vi "NIVEL DE TANQUE.vi"() -> ()   [LabVIEW 2019]
panel:
  in  "Velocidad de Llenado":dbl(knob) scale=0.0..10.0
  in  "Accion":bool
  in  "Vaciado/Llenado":bool
  in  "Velocidad":bool
  out "Tanque Vacio":bool
  out "Tanque LLeno":bool
  out "Paro":bool
  out "Vaciando":bool
  out "Llenando":bool
  out "Tanque":dbl(slide) scale=0.0..1000.0
  # "LLENAR"
  # "VACIAR"
  # "ALTA"
  # "CONTINUAR"
  # "PARAR"
  # "BAJA"
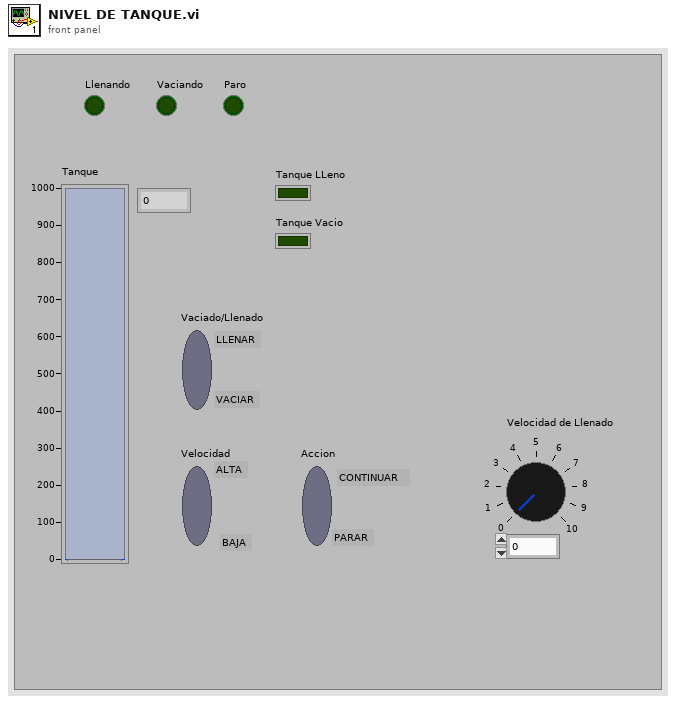
[diagram p1: front panel]
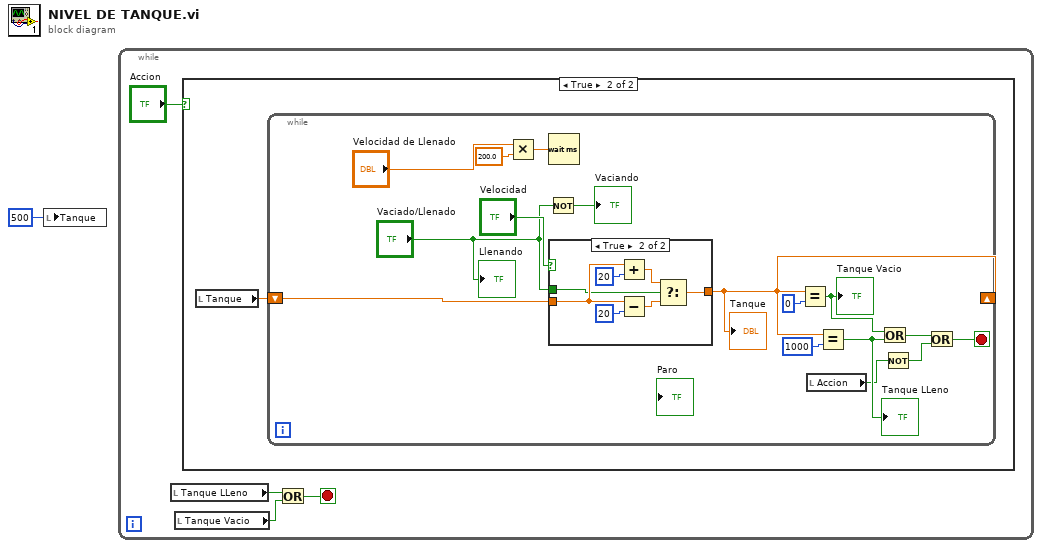
[diagram p0: block diagram]
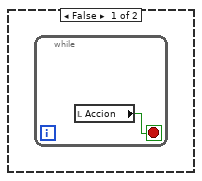
[diagram p2: hidden frame]
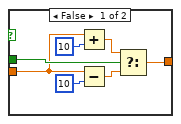
[diagram p3: hidden frame]
diagram:
  n1 = local write "Tanque"(500) -> ()
  n2 = while {
    stop <- w2 stop-if-true
    n3 = local read "Tanque LLeno"() -> (w4:bool)
    n4 = local read "Tanque Vacio"() -> (w3:bool)
    n5 = case shown="True" "Accion" {
      frame False {
        n6 = while {
          stop <- w6 stop-if-true
          n7 = local read "Accion"() -> (w6:bool)
        }
      }
      frame True {
        n8 = local read "Tanque"() -> (w7:dbl)
        n9 = while {
          shift-right: [w20] -> _
          shift-left: w7 -> [w23]
          stop <- w8 stop-if-true
          n10 = Multiply(x="Velocidad de Llenado", y=200.0) -> (x*y=w15:dbl)
          n11 = Not(x="Vaciado/Llenado") -> (.not. x?=→"Vaciando":bool)
          n12 = Wait (ms)(milliseconds to wait=w15) -> ()  [unwired: 1 out]
          n13 = case shown="True" "Velocidad" {
            tunnel: w23 -> [w24 w33]
            tunnel: [w25 w31] -> w20
            tunnel: "Vaciado/Llenado" -> [w26 w32]
            frame False {
              n14 = Add(x=w24, y=10) -> (x+y=w28:dbl)
              n15 = Subtract(x=w24, y=10) -> (x-y=w27:dbl)
              n16 = Select(t=w28, s=w26, f=w27) -> (s? t:f=w25:dbl)
            }
            frame True {
              n17 = Add(x=w33, y=20) -> (x+y=w35:dbl)
              n18 = Subtract(x=w33, y=20) -> (x-y=w34:dbl)
              n19 = Select(t=w35, s=w32, f=w34) -> (s? t:f=w31:dbl)
            }
          }
          "Tanque" <- w20
          n20 = Equal?(x=w20, y=0) -> (x = y?=w16:bool)
          "Tanque Vacio" <- w16
          n21 = local read "Accion"() -> (w11:bool)
          n22 = Equal?(x=w20, y=1000) -> (x = y?=w17:bool)
          "Tanque LLeno" <- w17
          n23 = Or(x=w16, y=w17) -> (x .or. y?=w9:bool)
          n24 = Not(x=w11) -> (.not. x?=w10:bool)
          n25 = Or(x=w9, y=w10) -> (x .or. y?=w8:bool)
          "Llenando" <- "Vaciado/Llenado"
        }
      }
    }
    n26 = Or(x=w4, y=w3) -> (x .or. y?=w2:bool)
  }
